vi "VI Server_Get TabControl Cluster_ArrayInput.vi"(7 "TabControl Labels[]":string[](array[string]), 8 "error in":errorcluster, 11 "VI Server Cluster":T1) -> (0 "error out":errorcluster, 3 "VI Server Cluster.OUT":T1)   [LabVIEW 2020, in "VI Server Toolkit LV2013.lvlib"]
doc: "Extracts control labels and references containing in a multiple tab controls and merges onto incoming VI server Cluster.\nThe tab controls labels should be arranged in a hierarchical order."
uses:
  VI Server Toolkit LV2013.lvlib
  VI Server_TypeDefs/VI Server_RefsCluster.ctl
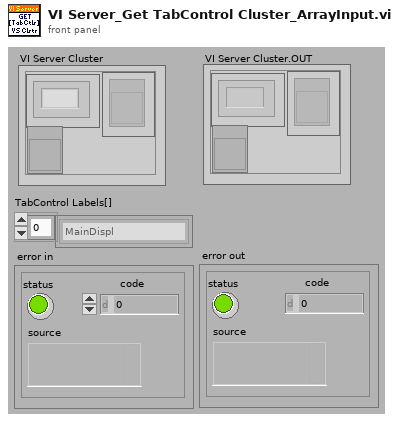
[diagram p1: front panel]
types:
  T1 = typedef "VI Server_RefsCluster.ctl" = cluster{"Labels":string[], "Refs":refnum<vi>[], "VI Ref":refnum<vi>}
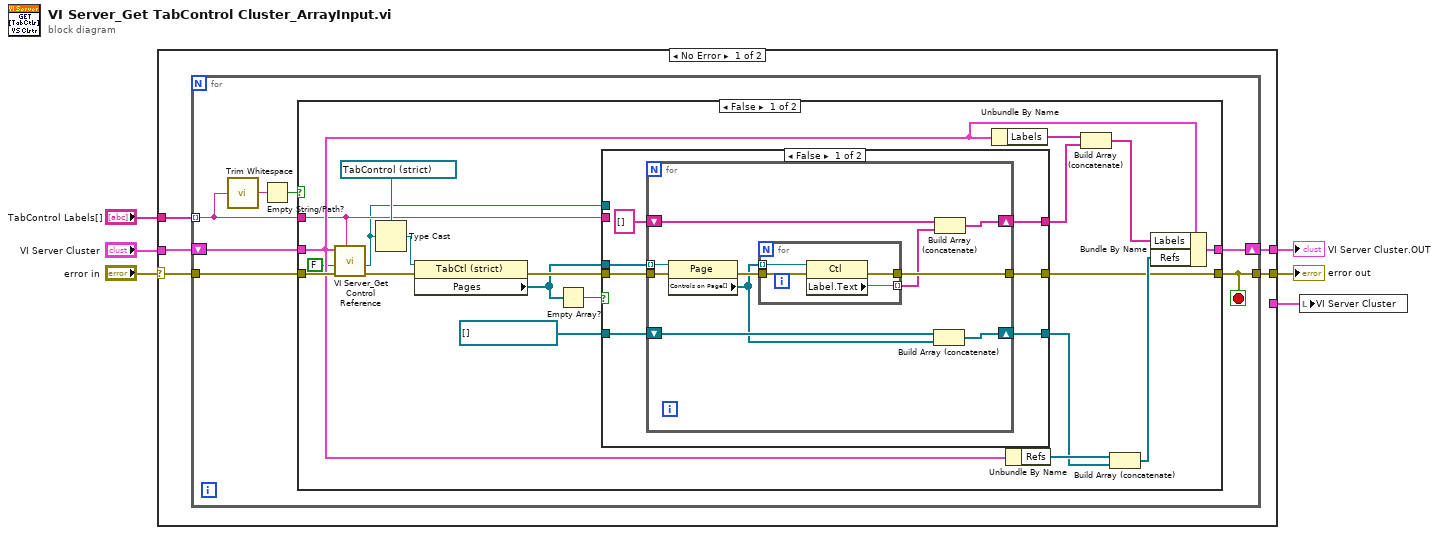
[diagram p0: block diagram]
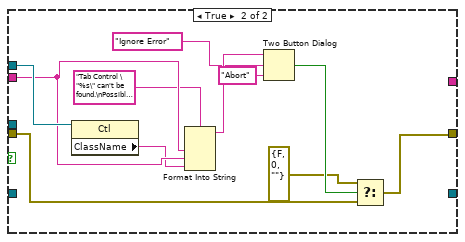
[diagram p2: hidden frame]
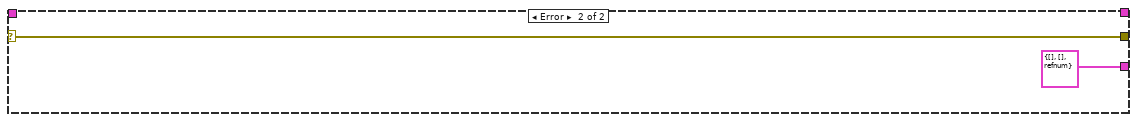
[diagram p4: hidden frame]
diagram:
  n1 = case shown="No Error" "error in" {
    selector: "error in" -> [w10 w74]
    tunnel: "VI Server Cluster" -> [w9 _]
    tunnel: [w11 w74] -> w5
    tunnel: "TabControl Labels[]" -> [w7 _]
    tunnel: [w8 _] -> w3
    tunnel: [_ T1 {"Labels"=[], "Refs"=[], "VI Ref"=refnum} ("VI Server Cluster")] -> w2
    frame No Error {
      n2 = for {
        tunnel: [w12] -> w11
        tunnel: w10 -> [w18]
        tunnel: w7 -> [w13] mode=indexing
        shift-right: [w14] -> w8
        shift-left: w9 -> [w17]
        stop <- w12 stop-if-true
        n3 = call <vilib>:"Trim Whitespace.vi"("string"=w13) -> ("trimmed string"=w16:string)  [unwired: 1 in]
        n4 = Empty String/Path?(string/path=w16) -> (empty?=w15:bool)
        n5 = case shown="False" w15 {
          tunnel: [w22 w72] -> w12
          tunnel: w18 -> [w38 w72]
          tunnel: w13 -> [w24 _]
          tunnel: w17 -> [w32 w71]
          tunnel: [w29 w71] -> w14
          frame False {
            n6 = call "VI Server_Get Control Reference.vi"("Label"=w24, "error in"=w38, "Single Instance (T)"=FALSE, "VI Server Cluster"=w32) -> ("error out"=w37:errorcluster, "Control Reference (Generic)"=w20:refnum<vi>)  [unwired: 6 out]
            n7 = Type Cast(type=refnum<vi> refnum ("TabCtlRef"), x=w20) -> (*(type *) &x=w21:refnum<vi>)
            n8 = property class="TabCtl (strict)"(reference=w21, error in=w37) -> (error out=w36:errorcluster, "Pages"=w26:refnum<vi>[])  [unwired: 1 out]
            n9 = Empty Array?(array=w26) -> (empty?=w25:bool)
            n10 = case shown="False" w25 {
              tunnel: [w45 w61] -> w22
              tunnel: w36 -> [w44 w62]
              tunnel: refnum<vi>[] [] ("Controls on Page[]") -> [w42 _]
              tunnel: [w41 _] -> w28
              tunnel: [w40 _] -> w23
              tunnel: w26 -> [w39 _]
              tunnel: w24 -> [_ w68]
              tunnel: w20 -> [_ w69]
              frame False {
                n11 = for {
                  tunnel: w44 -> [w54]
                  tunnel: [w52] -> w45
                  tunnel: w39 -> [w55] mode=indexing
                  shift-right: [w46] -> w40
                  shift-left: string[] [] -> [w51]
                  shift-right: [w48] -> w41
                  shift-left: w42 -> [w49]
                  n12 = property class="Page"(reference=w55, error in=w54) -> (error out=w53:errorcluster, "Controls on Page[]"=w47:refnum<vi>[])  [unwired: 1 out]
                  n13 = for {
                    tunnel: w53 -> [w59]
                    tunnel: w47 -> [w58] mode=indexing
                    tunnel: [w57] -> w52
                    tunnel: [w56] -> w50 mode=indexing
                    n14 = property class="Ctl"(reference=w58, error in=w59) -> (error out=w57:errorcluster, "Label.Text"=w56:string)  [unwired: 1 out]
                  }
                  n15 = Build Array (concatenate)(w49, w47) -> (w48:refnum<vi>[])
                  n16 = Build Array (concatenate)(w51, w50) -> (w46:string[])
                }
              }
              frame True {
                n17 = property class="Ctl"(reference=w69) -> ("ClassName"=w67:string)  [unwired: 1 in, 2 out]
                n18 = Format Into String(format string="Tab Control \"%s\" can't be found.\nPossible reason:\n1. Wrong name.\n2. It is part of another\nstacked structure.\n3. Control Label \"%s\" being entered for the tab is actually referencing to %s Class ID.", w68, w68, w67) -> (resulting string=w70:string)  [unwired: 2 in, 1 out]
                n19 = Two Button Dialog(message=w70, 1:"Abort" ("F button name (\"Cancel\")"), 2:"Ignore Error" ("T button name (\"OK\")")) -> (T button?=w63:bool)
                n20 = Select(t=errorcluster {"status"=FALSE, "code"=0, "source"=""}, s=w63, f=w62) -> (s? t:f=w61:errorcluster)
              }
            }
            n21 = Unbundle By Name(w32) -> ("Labels"=w34:string[])
            n22 = Unbundle By Name(w32) -> ("Refs"=w33:refnum<vi>[])
            n23 = Build Array (concatenate)(w34, w23) -> (w31:string[])
            n24 = Build Array (concatenate)(w33, w28) -> (w30:refnum<vi>[])
            n25 = Bundle By Name(cluster=w32, "Labels"=w31, "Refs"=w30) -> (w29:T1)
          }
          frame True {
          }
        }
      }
    }
    frame Error {
    }
  }
  "error out" <- w5
  "VI Server Cluster.OUT" <- w3
  n26 = local write "VI Server Cluster"(w2) -> ()
